vi "FIND DAQ Card.vi"(8 "Error In":errorcluster, 10 "Typ Karty":string="USB-6210") -> (0 "Error Out":errorcluster, 1 "Karta":T1, 2 "Znaleziono?":bool, 3 "DAQmx Device Name":tag, 4 "All Connected Devices":string[][](table))   [LabVIEW 2014]
doc: "Wyszukuje karty DAQ zainstalowane w systemie"
uses:
  Kontrolki/KartaDAQ/DAQ card Dane.ctl
  <resource>/objmgr/daqmx.rc
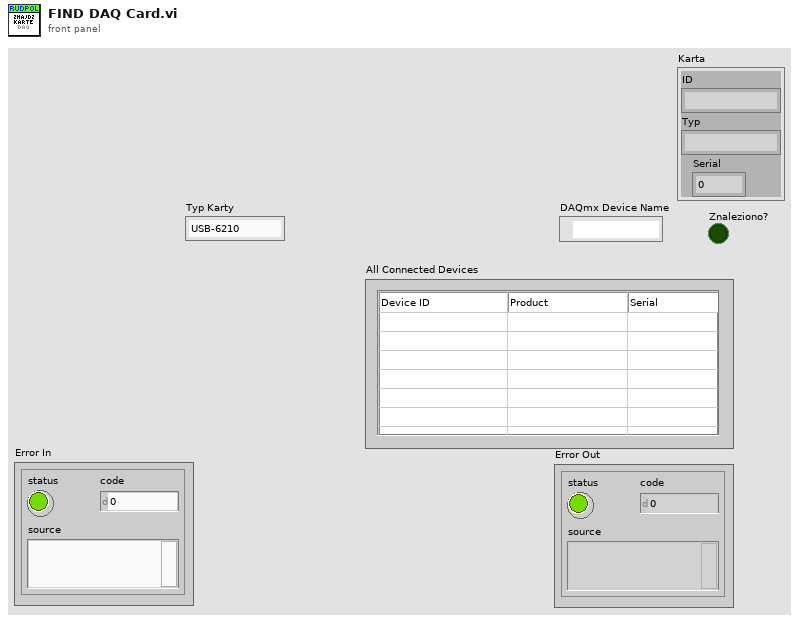
[diagram p1: front panel]
types:
  T1 = typedef "DAQ card Dane.ctl" = cluster{"ID":string, "Typ":string, "Serial":u32}
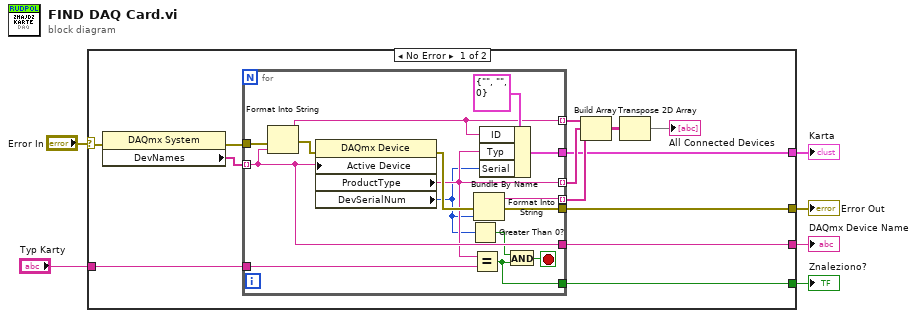
[diagram p0: block diagram]
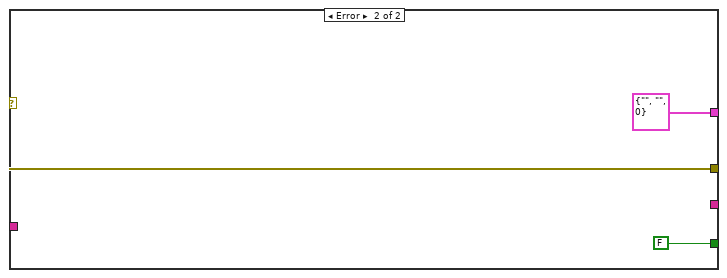
[diagram p2: hidden frame]
diagram:
  n1 = case shown="No Error" "Error In" {
    selector: "Error In" -> [w11 w37]
    tunnel: [w13 w37] -> w5
    tunnel: "Typ Karty" -> [w10 _]
    tunnel: [w9 T1 {"ID"="", "Typ"="", "Serial"=0}] -> w1
    tunnel: [w8 _] -> w3
    tunnel: [w7 FALSE] -> w2
    frame No Error {
      n2 = property class="DAQmx System"(error in=w11) -> (error out=w12:errorcluster, "DevNames"=w15:tag[])  [unwired: 1 in, 1 out]
      n3 = for {
        tunnel: w15 -> [w28] mode=indexing
        tunnel: [w22] -> w16 mode=indexing
        tunnel: [w23] -> w17 mode=indexing
        tunnel: [w34] -> w18 mode=indexing
        tunnel: [w31] -> w13
        tunnel: w12 -> [w30]
        tunnel: w10 -> [w29]
        tunnel: [w28] -> w8
        tunnel: [w26] -> w7
        tunnel: [w21] -> w9
        stop <- w27 stop-if-true
        n4 = Format Into String(error in=w30, w28) -> (resulting string=w23:string, error out=w33:errorcluster)  [unwired: 2 in]
        n5 = property class="DAQmx Device"(error in=w33, "Active Device"=w28) -> (error out=w32:errorcluster, "ProductType"=w22:string, "DevSerialNum"=w20:u32)  [unwired: 1 in, 1 out]
        n6 = Greater Than 0?(x=w20) -> (x > 0?=w25:bool)
        n7 = Equal?(x=w22, y=w29) -> (x = y?=w26:bool)
        n8 = Format Into String(error in=w32, w20) -> (resulting string=w34:string, error out=w31:errorcluster)  [unwired: 2 in]
        n9 = Bundle By Name(cluster=T1 {"ID"="", "Typ"="", "Serial"=0}, "ID"=w23, "Typ"=w22, "Serial"=w20) -> (w21:T1)
        n10 = And(x=w25, y=w26) -> (x .and. y?=w27:bool)
      }
      n11 = Build Array(w17, w16, w18) -> (w19:string[][])
      n12 = Transpose 2D Array(2D array=w19) -> (transposed array=→"All Connected Devices":string[][])
    }
    frame Error {
    }
  }
  "Error Out" <- w5
  "DAQmx Device Name" <- w3
  "Znaleziono?" <- w2
  "Karta" <- w1
